vi "Test Failing.vi"() -> ()   [LabVIEW 2020, in "Failing Test Case.lvclass"]
doc: "Failing test"
uses:
  Failing Test Case.lvclass
  C:/git/astemes-lunit/source/Core/LUnit Test Case/LUnit Test Case.lvclass
  LUnit Test Case.lvclass/LUnit Test Case.ctl
  Core/LUnit Test Case/Private/Append Fail Result.vi
  Core/LUnit Test Case/Private/Append Pass Result.vi
  Core/LUnit Test Case/Private/Run In UI.vi
  <vilib>/Utility/error.llb/Clear Errors.vi
  LUnit Test Case.lvclass
panel:
  out "Passing Test Case Out":refnum<class "Failing Test Case.lvclass">
  in  "Passing Test Case In":refnum<class "Failing Test Case.lvclass">
  out "error out":errorcluster
  in  "error in (no error)":errorcluster
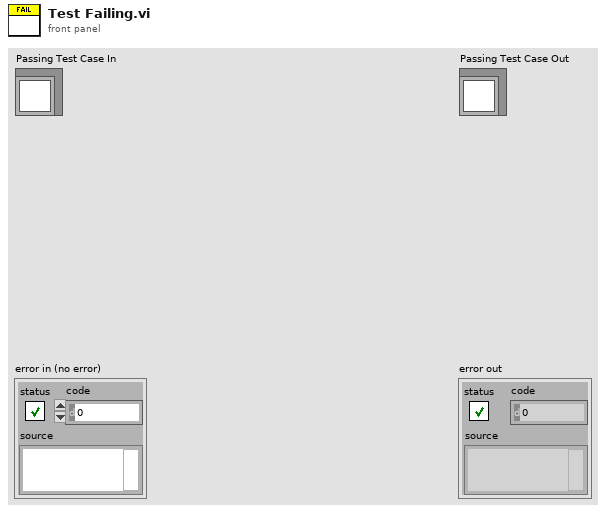
[diagram p1: front panel]
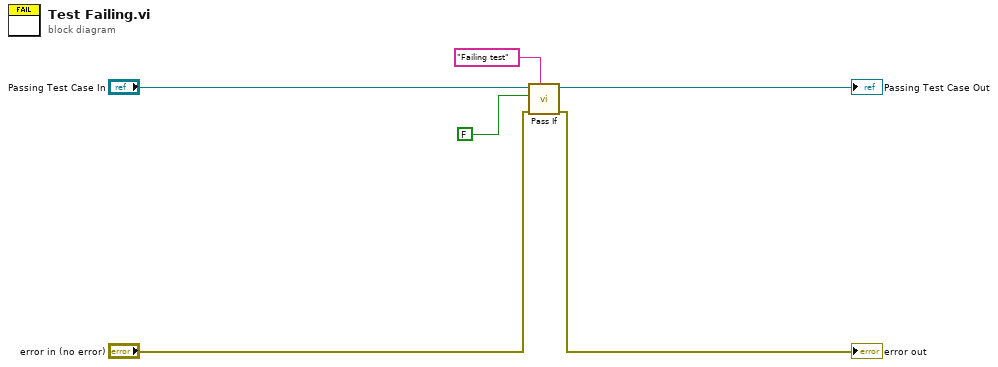
[diagram p0: block diagram]
diagram:
  n1 = call "Pass If.vi"("Description"="Failing test", "error in (no error)"="error in (no error)", "Pass?"=FALSE, "LUnit Test Case In"="Passing Test Case In") -> ("error out"=→"error out":errorcluster, "LUnit Test Case Out"=→"Passing Test Case Out":refnum<class "Failing Test Case.lvclass">)  [unwired: 6 in]
